vi "initialize_fifos_noSCTL_slow.vi"() -> (2 "Output State":i16)   [LabVIEW 2013]
uses:
  <vilib>/rvi/FIFO/Fifo_Resource/nirvififoEmulationGetNumberOfElementsToWriteFpgaImpl.vi
  <vilib>/rvi/DataTransferAndStorage/Container/Common/niFpgaContainerGetUniqueNameForEmu.vi
  <vilib>/rvi/FIFO/Fifo_Resource/nirvififoEmulationWriteFpgaImpl.vi
  <vilib>/rvi/DataTransferAndStorage/Container/XNode/niFpgaContainer.xnode
  <vilib>/rvi/FIFO/Fifo_Resource/nirvififoEmulationGetNumberOfElementsToWrite.vi
  <vilib>/rvi/FIFO/Fifo_Resource/nirvififoEmulationWrite.vi
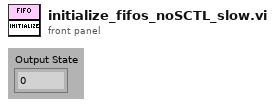
[diagram p1: front panel]
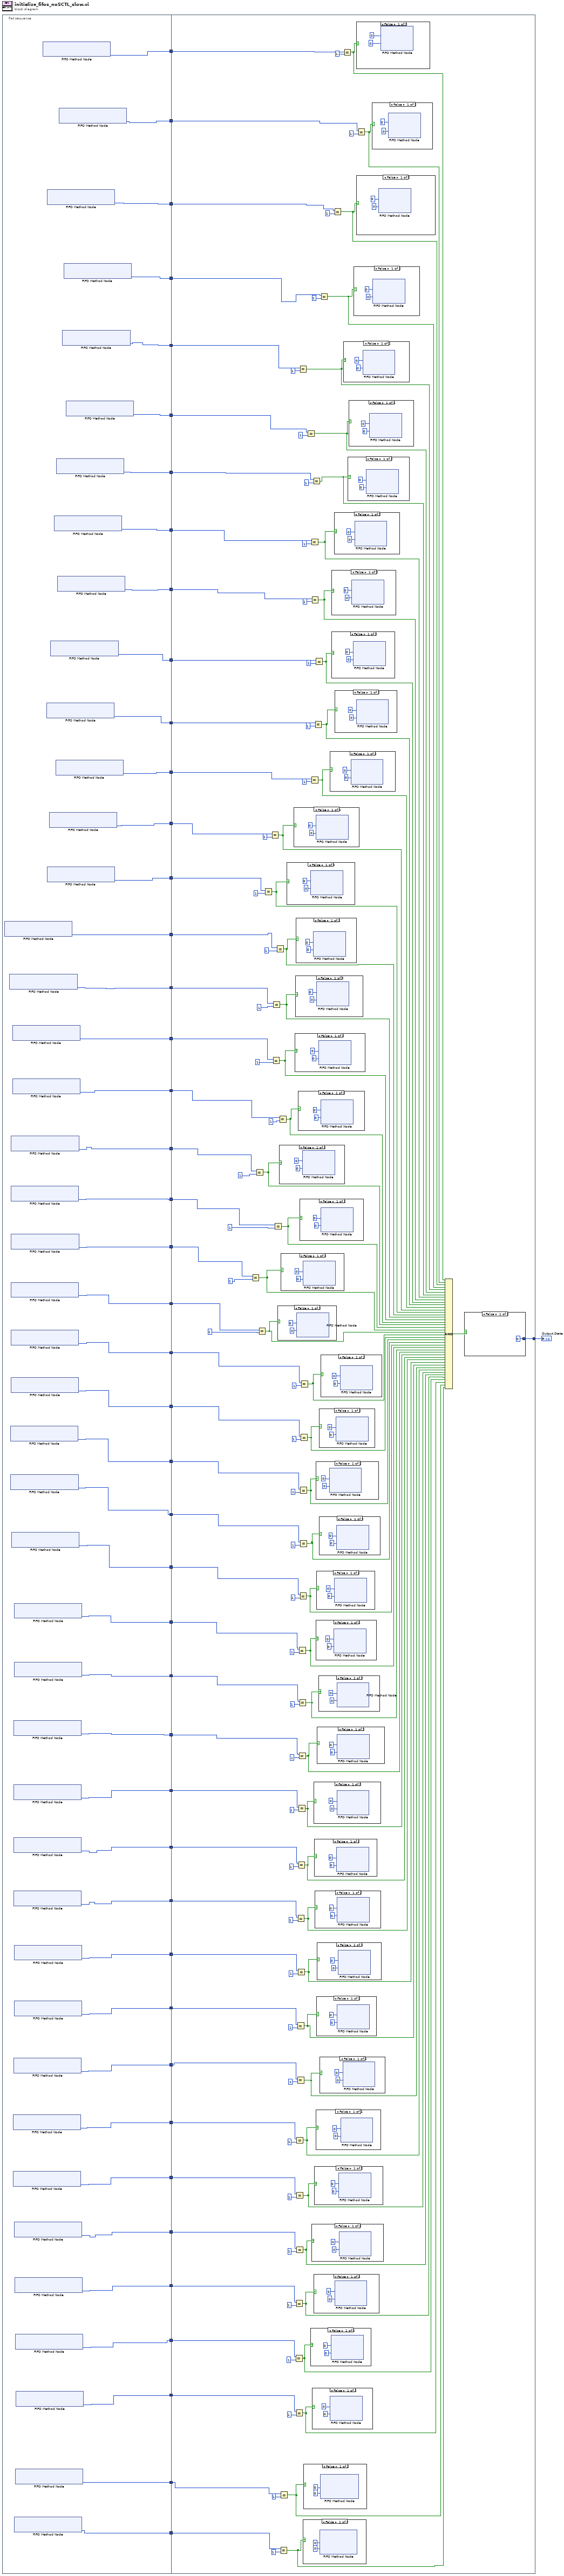
[diagram p0: block diagram]
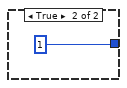
[diagram p3: hidden frame]
diagram:
  n1 = flat-sequence {
    tunnel: [w88] -> w45
    tunnel: [w87] -> w44
    tunnel: [w86] -> w43
    tunnel: [w85] -> w42
    tunnel: [w84] -> w41
    tunnel: [w83] -> w40
    tunnel: [w82] -> w39
    tunnel: [w81] -> w38
    tunnel: [w80] -> w37
    tunnel: [w79] -> w36
    tunnel: [w78] -> w35
    tunnel: [w77] -> w34
    tunnel: [w76] -> w33
    tunnel: [w75] -> w32
    tunnel: [w74] -> w31
    tunnel: [w73] -> w30
    tunnel: [w72] -> w29
    tunnel: [w71] -> w28
    tunnel: [w70] -> w27
    tunnel: [w69] -> w26
    tunnel: [w68] -> w25
    tunnel: [w67] -> w24
    tunnel: [w66] -> w23
    tunnel: [w65] -> w22
    tunnel: [w64] -> w21
    tunnel: [w63] -> w20
    tunnel: [w62] -> w19
    tunnel: [w61] -> w18
    tunnel: [w60] -> w17
    tunnel: [w59] -> w16
    tunnel: [w58] -> w15
    tunnel: [w57] -> w14
    tunnel: [w56] -> w13
    tunnel: [w55] -> w12
    tunnel: [w54] -> w11
    tunnel: [w53] -> w10
    tunnel: [w52] -> w9
    tunnel: [w51] -> w8
    tunnel: [w50] -> w7
    tunnel: [w49] -> w6
    tunnel: [w48] -> w5
    tunnel: [w47] -> w4
    tunnel: [w89] -> w3
    tunnel: [w46] -> w1
    tunnel: w45 -> [w223]
    tunnel: w44 -> [w222]
    tunnel: w43 -> [w221]
    tunnel: w42 -> [w220]
    tunnel: w41 -> [w219]
    tunnel: w40 -> [w218]
    tunnel: w39 -> [w217]
    tunnel: w38 -> [w216]
    tunnel: w37 -> [w215]
    tunnel: w36 -> [w214]
    tunnel: w35 -> [w213]
    tunnel: w34 -> [w212]
    tunnel: w33 -> [w211]
    tunnel: w32 -> [w210]
    tunnel: w31 -> [w209]
    tunnel: w30 -> [w208]
    tunnel: w29 -> [w207]
    tunnel: w28 -> [w206]
    tunnel: w27 -> [w205]
    tunnel: w26 -> [w204]
    tunnel: w25 -> [w203]
    tunnel: w24 -> [w202]
    tunnel: w23 -> [w201]
    tunnel: w22 -> [w200]
    tunnel: w21 -> [w199]
    tunnel: w20 -> [w198]
    tunnel: w19 -> [w197]
    tunnel: w18 -> [w196]
    tunnel: w17 -> [w195]
    tunnel: w16 -> [w194]
    tunnel: w15 -> [w193]
    tunnel: w14 -> [w192]
    tunnel: w13 -> [w191]
    tunnel: w12 -> [w190]
    tunnel: w11 -> [w189]
    tunnel: w10 -> [w188]
    tunnel: w9 -> [w187]
    tunnel: w8 -> [w186]
    tunnel: w7 -> [w185]
    tunnel: w6 -> [w184]
    tunnel: w5 -> [w183]
    tunnel: w4 -> [w182]
    tunnel: w3 -> [w181]
    tunnel: [w93] -> w2
    tunnel: w1 -> [w91]
    frame #0 {
      n2 = xnode ("FIFO Method Node")() -> ("Number of Elements to Write"=w74:u32)  [unwired: 1 in, 1 out]
      n3 = xnode ("FIFO Method Node")() -> ("Number of Elements to Write"=w73:u32)  [unwired: 1 in, 1 out]
      n4 = xnode ("FIFO Method Node")() -> ("Number of Elements to Write"=w64:u32)  [unwired: 1 in, 1 out]
      n5 = xnode ("FIFO Method Node")() -> ("Number of Elements to Write"=w63:u32)  [unwired: 1 in, 1 out]
      n6 = xnode ("FIFO Method Node")() -> ("Number of Elements to Write"=w69:u32)  [unwired: 1 in, 1 out]
      n7 = xnode ("FIFO Method Node")() -> ("Number of Elements to Write"=w67:u32)  [unwired: 1 in, 1 out]
      n8 = xnode ("FIFO Method Node")() -> ("Number of Elements to Write"=w66:u32)  [unwired: 1 in, 1 out]
      n9 = xnode ("FIFO Method Node")() -> ("Number of Elements to Write"=w65:u32)  [unwired: 1 in, 1 out]
      n10 = xnode ("FIFO Method Node")() -> ("Number of Elements to Write"=w70:u32)  [unwired: 1 in, 1 out]
      n11 = xnode ("FIFO Method Node")() -> ("Number of Elements to Write"=w68:u32)  [unwired: 1 in, 1 out]
      n12 = xnode ("FIFO Method Node")() -> ("Number of Elements to Write"=w62:u32)  [unwired: 1 in, 1 out]
      n13 = xnode ("FIFO Method Node")() -> ("Number of Elements to Write"=w72:u32)  [unwired: 1 in, 1 out]
      n14 = xnode ("FIFO Method Node")() -> ("Number of Elements to Write"=w71:u32)  [unwired: 1 in, 1 out]
      n15 = xnode ("FIFO Method Node")() -> ("Number of Elements to Write"=w52:u32)  [unwired: 1 in, 1 out]
      n16 = xnode ("FIFO Method Node")() -> ("Number of Elements to Write"=w51:u32)  [unwired: 1 in, 1 out]
      n17 = xnode ("FIFO Method Node")() -> ("Number of Elements to Write"=w59:u32)  [unwired: 1 in, 1 out]
      n18 = xnode ("FIFO Method Node")() -> ("Number of Elements to Write"=w58:u32)  [unwired: 1 in, 1 out]
      n19 = xnode ("FIFO Method Node")() -> ("Number of Elements to Write"=w57:u32)  [unwired: 1 in, 1 out]
      n20 = xnode ("FIFO Method Node")() -> ("Number of Elements to Write"=w56:u32)  [unwired: 1 in, 1 out]
      n21 = xnode ("FIFO Method Node")() -> ("Number of Elements to Write"=w53:u32)  [unwired: 1 in, 1 out]
      n22 = xnode ("FIFO Method Node")() -> ("Number of Elements to Write"=w61:u32)  [unwired: 1 in, 1 out]
      n23 = xnode ("FIFO Method Node")() -> ("Number of Elements to Write"=w60:u32)  [unwired: 1 in, 1 out]
      n24 = xnode ("FIFO Method Node")() -> ("Number of Elements to Write"=w55:u32)  [unwired: 1 in, 1 out]
      n25 = xnode ("FIFO Method Node")() -> ("Number of Elements to Write"=w54:u32)  [unwired: 1 in, 1 out]
      n26 = xnode ("FIFO Method Node")() -> ("Number of Elements to Write"=w50:u32)  [unwired: 1 in, 1 out]
      n27 = xnode ("FIFO Method Node")() -> ("Number of Elements to Write"=w46:u32)  [unwired: 1 in, 1 out]
      n28 = xnode ("FIFO Method Node")() -> ("Number of Elements to Write"=w49:u32)  [unwired: 1 in, 1 out]
      n29 = xnode ("FIFO Method Node")() -> ("Number of Elements to Write"=w48:u32)  [unwired: 1 in, 1 out]
      n30 = xnode ("FIFO Method Node")() -> ("Number of Elements to Write"=w89:u32)  [unwired: 1 in, 1 out]
      n31 = xnode ("FIFO Method Node")() -> ("Number of Elements to Write"=w47:u32)  [unwired: 1 in, 1 out]
      n32 = xnode ("FIFO Method Node")() -> ("Number of Elements to Write"=w88:u32)  [unwired: 1 in, 1 out]
      n33 = xnode ("FIFO Method Node")() -> ("Number of Elements to Write"=w78:u32)  [unwired: 1 in, 1 out]
      n34 = xnode ("FIFO Method Node")() -> ("Number of Elements to Write"=w75:u32)  [unwired: 1 in, 1 out]
      n35 = xnode ("FIFO Method Node")() -> ("Number of Elements to Write"=w86:u32)  [unwired: 1 in, 1 out]
      n36 = xnode ("FIFO Method Node")() -> ("Number of Elements to Write"=w76:u32)  [unwired: 1 in, 1 out]
      n37 = xnode ("FIFO Method Node")() -> ("Number of Elements to Write"=w79:u32)  [unwired: 1 in, 1 out]
      n38 = xnode ("FIFO Method Node")() -> ("Number of Elements to Write"=w81:u32)  [unwired: 1 in, 1 out]
      n39 = xnode ("FIFO Method Node")() -> ("Number of Elements to Write"=w77:u32)  [unwired: 1 in, 1 out]
      n40 = xnode ("FIFO Method Node")() -> ("Number of Elements to Write"=w82:u32)  [unwired: 1 in, 1 out]
      n41 = xnode ("FIFO Method Node")() -> ("Number of Elements to Write"=w80:u32)  [unwired: 1 in, 1 out]
      n42 = xnode ("FIFO Method Node")() -> ("Number of Elements to Write"=w87:u32)  [unwired: 1 in, 1 out]
      n43 = xnode ("FIFO Method Node")() -> ("Number of Elements to Write"=w84:u32)  [unwired: 1 in, 1 out]
      n44 = xnode ("FIFO Method Node")() -> ("Number of Elements to Write"=w85:u32)  [unwired: 1 in, 1 out]
      n45 = xnode ("FIFO Method Node")() -> ("Number of Elements to Write"=w83:u32)  [unwired: 1 in, 1 out]
    }
    frame #1 {
      n46 = Equal?(x=w203, y=u32 1) -> (x = y?=w117:bool)
      n47 = Equal?(x=w205, y=u32 1) -> (x = y?=w119:bool)
      n48 = Equal?(x=w202, y=u32 1) -> (x = y?=w116:bool)
      n49 = Equal?(x=w210, y=u32 1) -> (x = y?=w124:bool)
      n50 = Equal?(x=w211, y=u32 1) -> (x = y?=w125:bool)
      n51 = Equal?(x=w207, y=u32 1) -> (x = y?=w121:bool)
      n52 = Equal?(x=w208, y=u32 1) -> (x = y?=w122:bool)
      n53 = Equal?(x=w204, y=u32 1) -> (x = y?=w118:bool)
      n54 = Equal?(x=w209, y=u32 1) -> (x = y?=w123:bool)
      n55 = case shown="False" w116 {
        frame False {
          n56 = xnode ("FIFO Method Node")("Element"=0, "Timeout"=0) -> ()  [unwired: 1 in, 2 out]
        }
        frame True {
        }
      }
      n57 = Equal?(x=w206, y=u32 1) -> (x = y?=w120:bool)
      n58 = Equal?(x=w91, y=u32 1) -> (x = y?=w90:bool)
      n59 = case shown="False" w119 {
        frame False {
          n60 = xnode ("FIFO Method Node")("Element"=0, "Timeout"=0) -> ()  [unwired: 1 in, 2 out]
        }
        frame True {
        }
      }
      n61 = Equal?(x=w181, y=u32 1) -> (x = y?=w95:bool)
      n62 = case shown="False" w117 {
        frame False {
          n63 = xnode ("FIFO Method Node")("Element"=0, "Timeout"=0) -> ()  [unwired: 1 in, 2 out]
        }
        frame True {
        }
      }
      n64 = case shown="False" w124 {
        frame False {
          n65 = xnode ("FIFO Method Node")("Element"=0, "Timeout"=0) -> ()  [unwired: 1 in, 2 out]
        }
        frame True {
        }
      }
      n66 = case shown="False" w125 {
        frame False {
          n67 = xnode ("FIFO Method Node")("Element"=0, "Timeout"=0) -> ()  [unwired: 1 in, 2 out]
        }
        frame True {
        }
      }
      n68 = Equal?(x=w183, y=u32 1) -> (x = y?=w97:bool)
      n69 = Equal?(x=w184, y=u32 1) -> (x = y?=w98:bool)
      n70 = Equal?(x=w182, y=u32 1) -> (x = y?=w96:bool)
      n71 = case shown="False" w121 {
        frame False {
          n72 = xnode ("FIFO Method Node")("Element"=0, "Timeout"=0) -> ()  [unwired: 1 in, 2 out]
        }
        frame True {
        }
      }
      n73 = Equal?(x=w187, y=u32 1) -> (x = y?=w101:bool)
      n74 = Equal?(x=w186, y=u32 1) -> (x = y?=w100:bool)
      n75 = Equal?(x=w185, y=u32 1) -> (x = y?=w99:bool)
      n76 = case shown="False" w122 {
        frame False {
          n77 = xnode ("FIFO Method Node")("Element"=0, "Timeout"=0) -> ()  [unwired: 1 in, 2 out]
        }
        frame True {
        }
      }
      n78 = case shown="False" w123 {
        frame False {
          n79 = xnode ("FIFO Method Node")("Element"=0, "Timeout"=0) -> ()  [unwired: 1 in, 2 out]
        }
        frame True {
        }
      }
      n80 = Equal?(x=w189, y=u32 1) -> (x = y?=w103:bool)
      n81 = Equal?(x=w188, y=u32 1) -> (x = y?=w102:bool)
      n82 = Equal?(x=w191, y=u32 1) -> (x = y?=w105:bool)
      n83 = Equal?(x=w190, y=u32 1) -> (x = y?=w104:bool)
      n84 = Equal?(x=w192, y=u32 1) -> (x = y?=w106:bool)
      n85 = Equal?(x=w193, y=u32 1) -> (x = y?=w107:bool)
      n86 = Equal?(x=w196, y=u32 1) -> (x = y?=w110:bool)
      n87 = Equal?(x=w194, y=u32 1) -> (x = y?=w108:bool)
      n88 = Equal?(x=w195, y=u32 1) -> (x = y?=w109:bool)
      n89 = case shown="False" w120 {
        frame False {
          n90 = xnode ("FIFO Method Node")("Element"=0, "Timeout"=0) -> ()  [unwired: 1 in, 2 out]
        }
        frame True {
        }
      }
      n91 = Equal?(x=w219, y=u32 1) -> (x = y?=w133:bool)
      n92 = Equal?(x=w197, y=u32 1) -> (x = y?=w111:bool)
      n93 = Equal?(x=w199, y=u32 1) -> (x = y?=w113:bool)
      n94 = Equal?(x=w198, y=u32 1) -> (x = y?=w112:bool)
      n95 = Equal?(x=w200, y=u32 1) -> (x = y?=w114:bool)
      n96 = case shown="False" w118 {
        frame False {
          n97 = xnode ("FIFO Method Node")("Element"=0, "Timeout"=0) -> ()  [unwired: 1 in, 2 out]
        }
        frame True {
        }
      }
      n98 = Equal?(x=w201, y=u32 1) -> (x = y?=w115:bool)
      n99 = case shown="False" w90 {
        frame False {
          n100 = xnode ("FIFO Method Node")("Element"=0, "Timeout"=0) -> ()  [unwired: 1 in, 2 out]
        }
        frame True {
        }
      }
      n101 = case shown="False" w95 {
        frame False {
          n102 = xnode ("FIFO Method Node")("Element"=0, "Timeout"=0) -> ()  [unwired: 1 in, 2 out]
        }
        frame True {
        }
      }
      n103 = Equal?(x=w218, y=u32 1) -> (x = y?=w132:bool)
      n104 = Equal?(x=w216, y=u32 1) -> (x = y?=w130:bool)
      n105 = Equal?(x=w212, y=u32 1) -> (x = y?=w126:bool)
      n106 = Equal?(x=w215, y=u32 1) -> (x = y?=w129:bool)
      n107 = case shown="False" w97 {
        frame False {
          n108 = xnode ("FIFO Method Node")("Element"=0, "Timeout"=0) -> ()  [unwired: 1 in, 2 out]
        }
        frame True {
        }
      }
      n109 = Equal?(x=w217, y=u32 1) -> (x = y?=w131:bool)
      n110 = case shown="False" w99 {
        frame False {
          n111 = xnode ("FIFO Method Node")("Element"=0, "Timeout"=0) -> ()  [unwired: 1 in, 2 out]
        }
        frame True {
        }
      }
      n112 = case shown="False" w96 {
        frame False {
          n113 = xnode ("FIFO Method Node")("Element"=0, "Timeout"=0) -> ()  [unwired: 1 in, 2 out]
        }
        frame True {
        }
      }
      n114 = Equal?(x=w213, y=u32 1) -> (x = y?=w127:bool)
      n115 = case shown="False" w107 {
        frame False {
          n116 = xnode ("FIFO Method Node")("Element"=0, "Timeout"=0) -> ()  [unwired: 1 in, 2 out]
        }
        frame True {
        }
      }
      n117 = case shown="False" w98 {
        frame False {
          n118 = xnode ("FIFO Method Node")("Element"=0, "Timeout"=0) -> ()  [unwired: 1 in, 2 out]
        }
        frame True {
        }
      }
      n119 = Equal?(x=w214, y=u32 1) -> (x = y?=w128:bool)
      n120 = case shown="False" w106 {
        frame False {
          n121 = xnode ("FIFO Method Node")("Element"=0, "Timeout"=0) -> ()  [unwired: 1 in, 2 out]
        }
        frame True {
        }
      }
      n122 = case shown="False" w100 {
        frame False {
          n123 = xnode ("FIFO Method Node")("Element"=0, "Timeout"=0) -> ()  [unwired: 1 in, 2 out]
        }
        frame True {
        }
      }
      n124 = case shown="False" w105 {
        frame False {
          n125 = xnode ("FIFO Method Node")("Element"=0, "Timeout"=0) -> ()  [unwired: 1 in, 2 out]
        }
        frame True {
        }
      }
      n126 = case shown="False" w113 {
        frame False {
          n127 = xnode ("FIFO Method Node")("Element"=0, "Timeout"=0) -> ()  [unwired: 1 in, 2 out]
        }
        frame True {
        }
      }
      n128 = case shown="False" w110 {
        frame False {
          n129 = xnode ("FIFO Method Node")("Element"=0, "Timeout"=0) -> ()  [unwired: 1 in, 2 out]
        }
        frame True {
        }
      }
      n130 = case shown="False" w101 {
        frame False {
          n131 = xnode ("FIFO Method Node")("Element"=0, "Timeout"=0) -> ()  [unwired: 1 in, 2 out]
        }
        frame True {
        }
      }
      n132 = case shown="False" w111 {
        frame False {
          n133 = xnode ("FIFO Method Node")("Element"=0, "Timeout"=0) -> ()  [unwired: 1 in, 2 out]
        }
        frame True {
        }
      }
      n134 = case shown="False" w103 {
        frame False {
          n135 = xnode ("FIFO Method Node")("Element"=0, "Timeout"=0) -> ()  [unwired: 1 in, 2 out]
        }
        frame True {
        }
      }
      n136 = case shown="False" w108 {
        frame False {
          n137 = xnode ("FIFO Method Node")("Element"=0, "Timeout"=0) -> ()  [unwired: 1 in, 2 out]
        }
        frame True {
        }
      }
      n138 = case shown="False" w104 {
        frame False {
          n139 = xnode ("FIFO Method Node")("Element"=0, "Timeout"=0) -> ()  [unwired: 1 in, 2 out]
        }
        frame True {
        }
      }
      n140 = case shown="False" w109 {
        frame False {
          n141 = xnode ("FIFO Method Node")("Element"=0, "Timeout"=0) -> ()  [unwired: 1 in, 2 out]
        }
        frame True {
        }
      }
      n142 = case shown="False" w114 {
        frame False {
          n143 = xnode ("FIFO Method Node")("Element"=0, "Timeout"=0) -> ()  [unwired: 1 in, 2 out]
        }
        frame True {
        }
      }
      n144 = case shown="False" w112 {
        frame False {
          n145 = xnode ("FIFO Method Node")("Element"=0, "Timeout"=0) -> ()  [unwired: 1 in, 2 out]
        }
        frame True {
        }
      }
      n146 = Equal?(x=w220, y=u32 1) -> (x = y?=w134:bool)
      n147 = case shown="False" w102 {
        frame False {
          n148 = xnode ("FIFO Method Node")("Element"=0, "Timeout"=0) -> ()  [unwired: 1 in, 2 out]
        }
        frame True {
        }
      }
      n149 = case shown="False" w115 {
        frame False {
          n150 = xnode ("FIFO Method Node")("Element"=0, "Timeout"=0) -> ()  [unwired: 1 in, 2 out]
        }
        frame True {
        }
      }
      n151 = case shown="False" w126 {
        frame False {
          n152 = xnode ("FIFO Method Node")("Element"=0, "Timeout"=0) -> ()  [unwired: 1 in, 2 out]
        }
        frame True {
        }
      }
      n153 = case shown="False" w129 {
        frame False {
          n154 = xnode ("FIFO Method Node")("Element"=0, "Timeout"=0) -> ()  [unwired: 1 in, 2 out]
        }
        frame True {
        }
      }
      n155 = case shown="False" w128 {
        frame False {
          n156 = xnode ("FIFO Method Node")("Element"=0, "Timeout"=0) -> ()  [unwired: 1 in, 2 out]
        }
        frame True {
        }
      }
      n157 = Equal?(x=w221, y=u32 1) -> (x = y?=w135:bool)
      n158 = case shown="False" w130 {
        frame False {
          n159 = xnode ("FIFO Method Node")("Element"=0, "Timeout"=0) -> ()  [unwired: 1 in, 2 out]
        }
        frame True {
        }
      }
      n160 = case shown="False" w127 {
        frame False {
          n161 = xnode ("FIFO Method Node")("Element"=0, "Timeout"=0) -> ()  [unwired: 1 in, 2 out]
        }
        frame True {
        }
      }
      n162 = Equal?(x=w223, y=u32 1) -> (x = y?=w137:bool)
      n163 = case shown="False" w133 {
        frame False {
          n164 = xnode ("FIFO Method Node")("Element"=0, "Timeout"=0) -> ()  [unwired: 1 in, 2 out]
        }
        frame True {
        }
      }
      n165 = case shown="False" w131 {
        frame False {
          n166 = xnode ("FIFO Method Node")("Element"=0, "Timeout"=0) -> ()  [unwired: 1 in, 2 out]
        }
        frame True {
        }
      }
      n167 = case shown="False" w132 {
        frame False {
          n168 = xnode ("FIFO Method Node")("Element"=0, "Timeout"=0) -> ()  [unwired: 1 in, 2 out]
        }
        frame True {
        }
      }
      n169 = case shown="False" w134 {
        frame False {
          n170 = xnode ("FIFO Method Node")("Element"=0, "Timeout"=0) -> ()  [unwired: 1 in, 2 out]
        }
        frame True {
        }
      }
      n171 = case shown="False" w137 {
        frame False {
          n172 = xnode ("FIFO Method Node")("Element"=0, "Timeout"=0) -> ()  [unwired: 1 in, 2 out]
        }
        frame True {
        }
      }
      n173 = Equal?(x=w222, y=u32 1) -> (x = y?=w136:bool)
      n174 = case shown="False" w135 {
        frame False {
          n175 = xnode ("FIFO Method Node")("Element"=0, "Timeout"=0) -> ()  [unwired: 1 in, 2 out]
        }
        frame True {
        }
      }
      n176 = case shown="False" w136 {
        frame False {
          n177 = xnode ("FIFO Method Node")("Element"=0, "Timeout"=0) -> ()  [unwired: 1 in, 2 out]
        }
        frame True {
        }
      }
      n178 = Compound Arithmetic op=AND(w137, w136, w135, w134, w133, w132, w131, w130, w129, w128, w127, w126, w125, w124, w123, w122, w121, w120, w119, w118, w117, w116, w115, w114, w113, w112, w111, w110, w109, w108, w107, w106, w105, w104, w103, w102, w101, w100, w99, w98, w97, w96, w95, w90) -> (w94:bool)
      n179 = case shown="False" w94 {
        tunnel: [i16 0 i16 1] -> w93
        frame False {
        }
        frame True {
        }
      }
    }
  }
  "Output State" <- w2
